vi "SubsystemModell.vi"(7 "Fk":dbl) -> (3 "p''":dbl, 4 "Postition":dbl, 6 "Geschwindigkeit":dbl, 8 "Winkel":dbl, 10 "p'":dbl, 14 "Beschleunigung":dbl)   [LabVIEW 2013]
uses:
  <vilib>/Simulation/Implementation/Shared/SIMSCR Execution Mode.ctl
  <vilib>/Simulation/Scripting/Companion Diagram/SimConfigNode/SimParams.ctl
  <vilib>/Simulation/Scripting/Companion Diagram/SimConfigNode/_simSolvers.ctl
  <vilib>/Simulation/Param Hierarchy/Typedefs/SIMPH Param Control Actions.ctl
  <vilib>/Simulation/Implementation/Shared/SIM limit type.ctl
  <vilib>/Simulation/Implementation/Shared/NILVSim_ParamChanged.vi
  <vilib>/Simulation/Implementation/Shared/NILVSIM_BeginStep.vi
  <vilib>/Simulation/ContinuousLinear/Implementation/NILVSim Integrator new.llb/SIM Integrator distributor (scalar).vi
  <vilib>/Simulation/SignalArithmetic/Implementation/NILVSim Gain.llb/SIM Gain (scalar).vi
  <vilib>/Simulation/ContinuousLinear/Implementation/NILVSim Integrator new.llb/SIM Integrator collector (scalar).vi
  <vilib>/Simulation/Implementation/Shared/NILVSim_Manager.vi
  <vilib>/Simulation/Implementation/Shared/NILVSim_FinalizeModel.vi
  <vilib>/Simulation/Implementation/Shared/SIM Unbundle Sim Info.vi
  <vilib>/Utility/error.llb/Clear Errors.vi
  <vilib>/Simulation/Implementation/Shared/NILVSim_GetModelError.vi
  <vilib>/Simulation/Implementation/Shared/SIM SimErrorHandler.vi
  <vilib>/Simulation/Implementation/Shared/SIM Bundle Sim Info.vi
  <vilib>/Simulation/Implementation/Shared/SIMSH Read Queue.vi
  Beschleunigung.vi
  geschwindigkeit.vi
  p''.vi
  p'.vi
  p.vi
  <vilib>/Simulation/Implementation/Shared/NILVSim_Initialize.vi
  <vilib>/Simulation/Utility/Implementation/NILVSim Get Time and IsAcceptedStep.vi
  <vilib>/Simulation/Scripting/Companion Diagram/SimConfigNode/SimDog.xnode
  <vilib>/Simulation/Implementation/XNodeFramework/SimXNode/SimX.xnode
  <vilib>/Simulation/ContinuousLinear/Implementation/NILVSim Integrator new.llb/SIM Integrator (scalar).vi
  <vilib>/Simulation/Implementation/Shared/NI_SIM_Implementation.lvlib
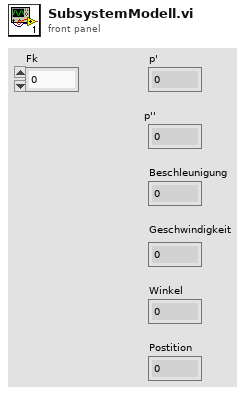
[diagram p1: front panel]
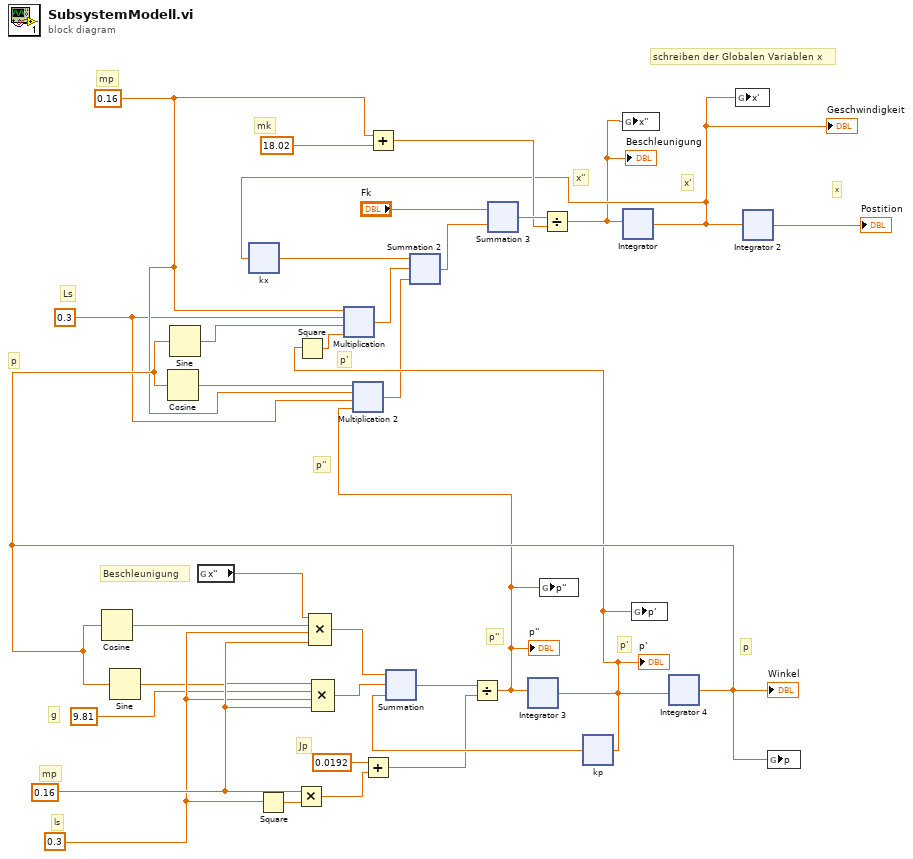
[diagram p0: block diagram]
diagram:
  w26 = 0.3 ("Constant 5")
  w27 = 0.16 ("Constant 4")
  w13 = 0.16 ("Constant 2")
  w12 = 0.3 ("Constant")
  # "schreiben der Globalen Variablen x"
  # "g"
  # "p''"
  # "Jp"
  # "Beschleunigung"
  # "ls"
  # "mp"
  # "p"
  # "p'"
  # "p''"
  # "mk"
  # "mp"
  # "Ls"
  # "p'"
  # "p"
  # "x"
  # "x'"
  # "x''"
  n1 = global read "Beschleunigung.vi 2" "x''"() -> (w30:dbl)
  n2 = Square ("Quadrat 2")(x=w26) -> (x^2=w18:dbl)
  n3 = Multiply ("Multiplizieren")(x=w27, y=w18) -> (x*y=w17:dbl)
  n4 = Add ("Addieren")(x=0.0192, y=w17) -> (x+y=w16:dbl)
  n5 = Add ("Addieren 2")(x=w13, y=18.02 ("Constant 3")) -> (x+y=w4:dbl)
  n6 = Cosine ("Cosinus 2")(x=w33) -> (cos(x)=w25:dbl)
  n7 = Compound Arithmetic op=MULTIPLY ("Mehrfacharithmetik")(w30, w25, w26, w27) -> (w20:dbl)
  n8 = Sine ("Sinus 2")(x=w33) -> (sin(x)=w22:dbl)
  n9 = Compound Arithmetic op=MULTIPLY ("Mehrfacharithmetik 2")(w22, 9.81 ("Wert"), w26, w27) -> (w21:dbl)
  n10 = Cosine ("Cosinus")(x=w33) -> (cos(x)=w10:dbl)
  n11 = Sine ("Sinus")(x=w33) -> (sin(x)=w6:dbl)
  n12 = xnode "kx"("input"=w3) -> ("output"=w5:dbl)  [unwired: 3 in]
  n13 = Square ("Quadrat")(x=w32) -> (x^2=w7:dbl)
  n14 = xnode ("Multiplication")("Operand1"=w13, "Operand2"=w12, "Operand3"=w6, "Operand4"=w7) -> ("Result"=w8:dbl)
  n15 = xnode ("Multiplication 2")("Operand1"=w10, "Operand2"=w13, "Operand3"=w12, "Operand4"=w31) -> ("Result"=w9:dbl)
  n16 = xnode ("Summation 2")("Operand1"=w5, "Operand2"=w8, "Operand3"=w9) -> ("Result"=w15:dbl)
  n17 = xnode ("Summation 3")("Operand1"="Fk", "Operand2"=w15) -> ("Result"=w11:dbl)
  n18 = Divide(x=w11, y=w4) -> (x/y=w2:dbl)
  "Beschleunigung" <- w2
  n19 = global write "Beschleunigung.vi" "x''"(w2) -> ()
  n20 = xnode ("Integrator")("input"=w2) -> ("output"=w3:dbl)  [unwired: 9 in, 2 out]
  "Geschwindigkeit" <- w3
  n21 = global write "geschwindigkeit.vi" "x'"(w3) -> ()
  n22 = xnode ("Integrator 2")("input"=w3) -> ("output"=→"Postition":dbl)  [unwired: 9 in, 2 out]
  n23 = xnode "Summation"("Operand1"=w20, "Operand2"=w21, "Operand3"=w24) -> ("Result"=w19:dbl)
  n24 = Divide ("Divide 2")(x=w19, y=w16) -> (x/y=w31:dbl)
  "p''" <- w31
  n25 = xnode ("Integrator 3")("input"=w31) -> ("output"=w32:dbl)  [unwired: 9 in, 2 out]
  "p'" <- w32
  n26 = global write "p''.vi 2" "p''"(w31) -> ()
  n27 = xnode "kp"("input"=w32) -> ("output"=w24:dbl)  [unwired: 3 in]
  n28 = global write "p'.vi 2" "p'"(w32) -> ()
  n29 = xnode ("Integrator 4")("input"=w32) -> ("output"=w33:dbl)  [unwired: 9 in, 2 out]
  "Winkel" <- w33
  n30 = global write "p.vi 2" "p"(w33) -> ()
